vi "Untitled 1.vi"() -> ()   [LabVIEW 2020]
panel:
  in  "Einzel":dbl(slide) scale=0.0..-10000.0
  in  "Anode":dbl(slide) scale=0.0..900.0
  in  "stop":bool
  out "einzel":dbl(graph)
  out "Einzel readback":dbl
  out "anode":dbl(graph)
  out "readback":dbl
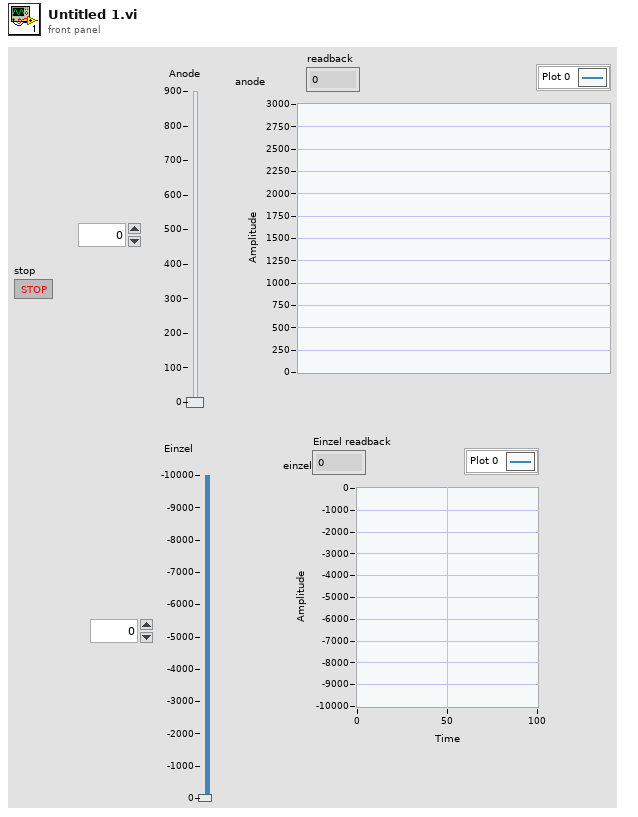
[diagram p1: front panel]
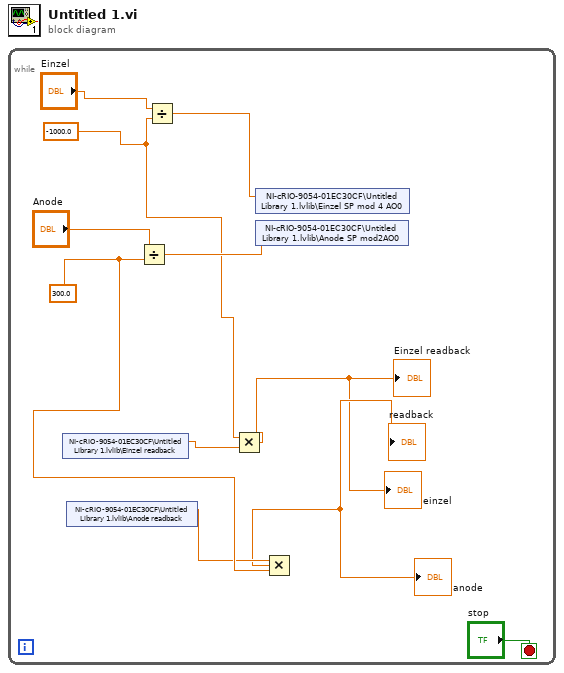
[diagram p0: block diagram]
diagram:
  n1 = while {
    stop <- "stop" stop-if-true
    w3 = -1000.0
    w6 = 300.0
    n2 = shared-variable "NI-cRIO-9054-01EC30CF\\Untitled Library 1.lvlib\\Einzel readback"() -> (w2:dbl)  [unwired: 1 in, 1 out]
    n3 = shared-variable "NI-cRIO-9054-01EC30CF\\Untitled Library 1.lvlib\\Anode readback"() -> (w5:dbl)  [unwired: 1 in, 1 out]
    n4 = Divide(x="Anode", y=w6) -> (x/y=w9:dbl)
    n5 = Divide(x="Einzel", y=w3) -> (x/y=w7:dbl)
    n6 = Multiply(x=w3, y=w2) -> (x*y=→"Einzel readback" →"einzel":dbl)
    n7 = shared-variable "NI-cRIO-9054-01EC30CF\\Untitled Library 1.lvlib\\Einzel SP mod 4 AO0"(w7) -> ()  [unwired: 1 in, 1 out]
    n8 = shared-variable "NI-cRIO-9054-01EC30CF\\Untitled Library 1.lvlib\\Anode SP mod2AO0"(w9) -> ()  [unwired: 1 in, 1 out]
    n9 = Multiply(x=w5, y=w6) -> (x*y=→"readback" →"anode":dbl)
  }
